vi "HXG2_SAVE Config File Values.vi"(8 "error in":errorcluster, 9 "BoolSelecOut":T1, 10 "AIR-GLY Cluster":T2 {"Liq Cluster"."Liq TEMP %" min=0.0 max=100.0 step=1.0 format="%#.1f"; "Liq Cluster"."Liq FLOW %" min=0.0 max=100.0 step=1.0 format="%#.1f"; "Liq Cluster"."TLiq °F" min=40.0 max=180.0 step=1.0 format="%#.1f"; "Liq Cluster"."Mdot lbm/hr" min=0.0 max=1000.0 step=1.0 format="%#.1f"; "Air Cluster"."Air TEMP %" min=0.0 max=100.0 step=1.0 format="%#.1f"; "Air Cluster"."Air FLOW %" min=0.0 max=100.0 step=1.0 format="%#.1f"; "Air Cluster"."Tair  °F" min=-5.0 max=100.0 step=1.0 format="%#.1f"; "Air Cluster"."CFMs" min=0.0 max=200.0 step=1.0 format="%#.1f"}) -> (0 "error out":errorcluster)   [LabVIEW 2012]
uses:
  Controls/HXG2_AirGly-Cluster.ctl
  Controls/UI/HXG2_UI_ControlSetAir.ctl
  Controls/UI/HXG2_UI_ControlSetGly.ctl
  Controls/HXG2_BooleanSelections.ctl
  <vilib>/Utility/file.llb/Write To Spreadsheet File (DBL).vi
panel:
  out "size(s)":i32
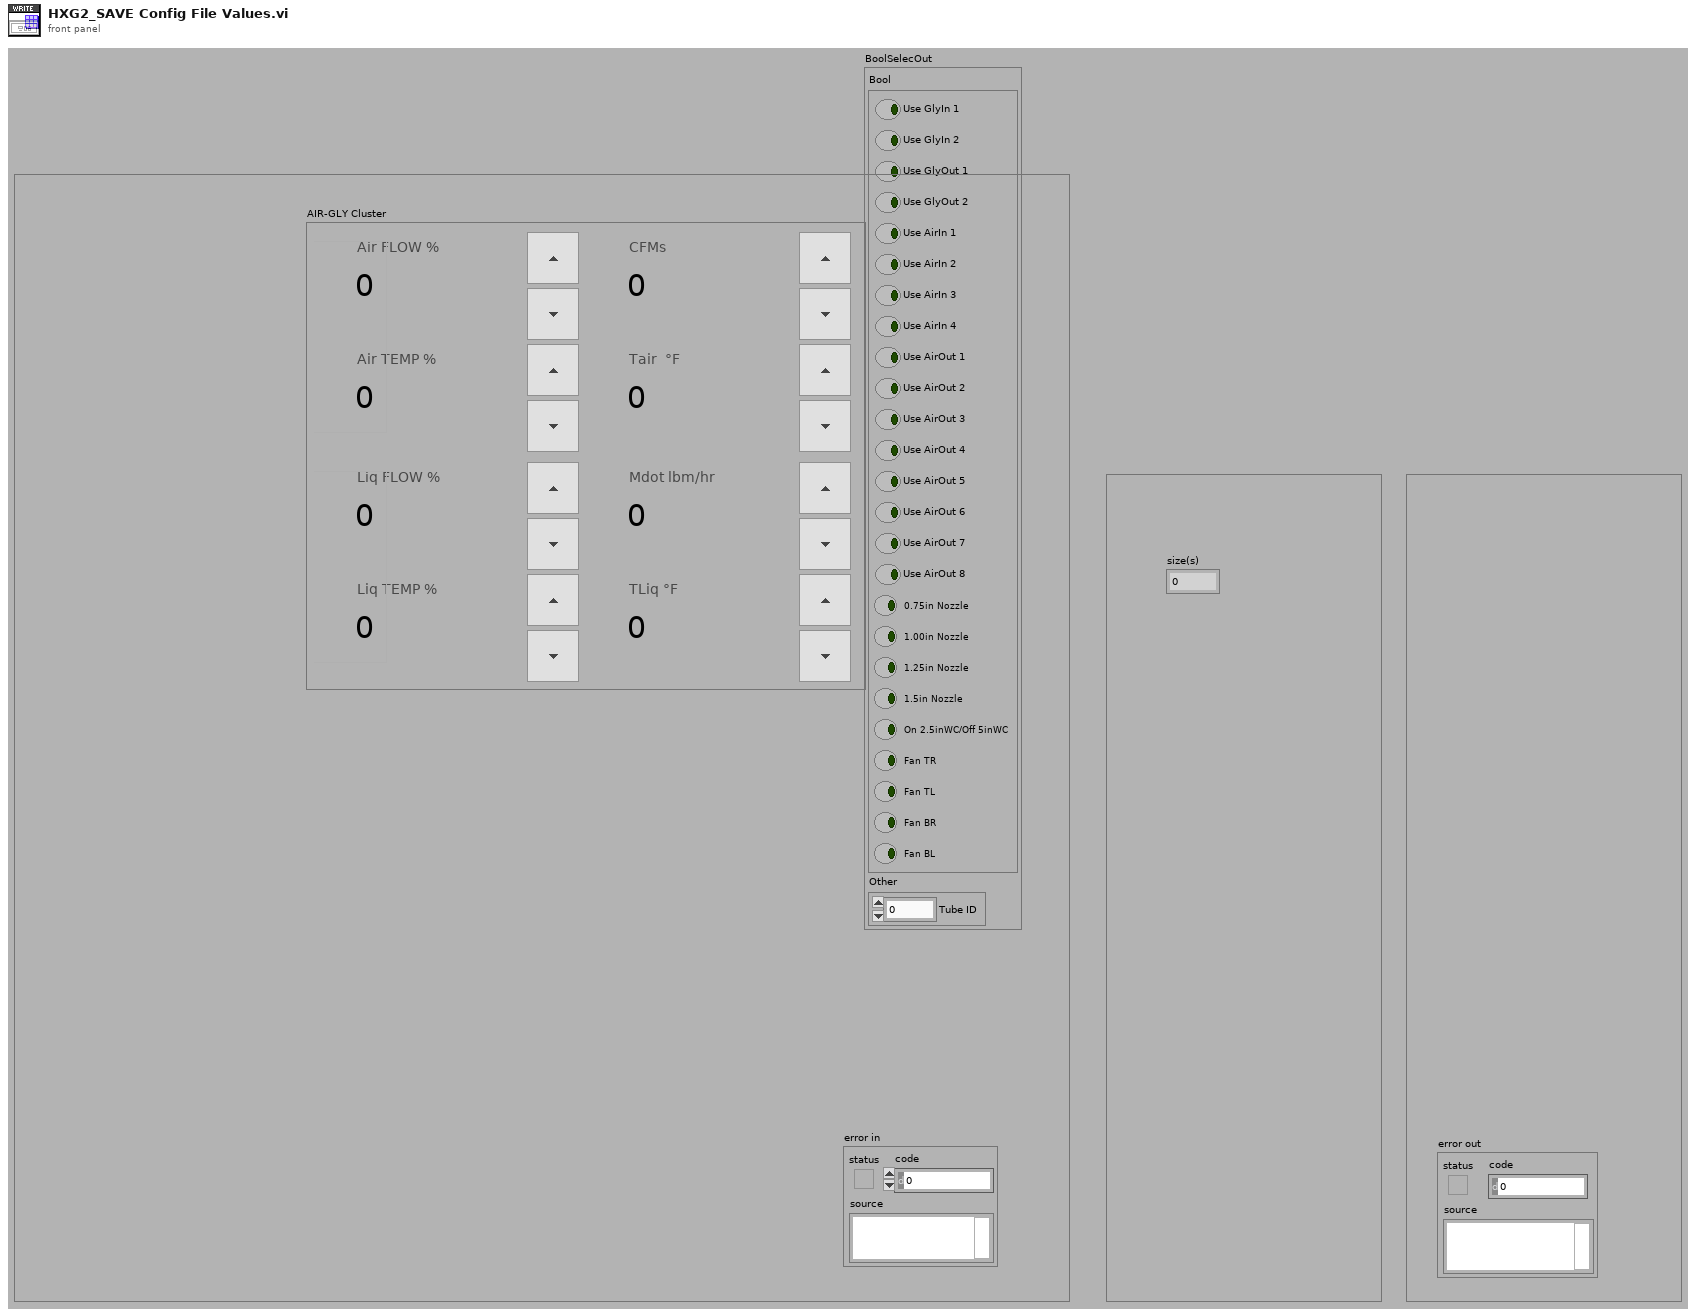
[diagram p1: front panel]
types:
  T1 = typedef "HXG2_BooleanSelections.ctl" = cluster{"Bool":cluster{"Use GlyIn 1":bool, "Use GlyIn 2":bool, "Use GlyOut 1":bool, "Use GlyOut 2":bool, "Use AirIn 1":bool, "Use AirIn 2":bool, "Use AirIn 3":bool, "Use AirIn 4":bool, "Use AirOut 1":bool, "Use AirOut 2":bool, "Use AirOut 3":bool, "Use AirOut 4":bool, "Use AirOut 5":bool, "Use AirOut 6":bool, "Use AirOut 7":bool, "Use AirOut 8":bool, "0.75in Nozzle":bool, "1.00in Nozzle":bool, "1.25in Nozzle":bool, "1.5in Nozzle":bool, "On 2.5inWC/Off 5inWC":bool, "Fan TR":bool, "Fan TL":bool, "Fan BR":bool, "Fan BL":bool}, "Other":cluster{"Tube ID":dbl}}
  T2 = typedef "HXG2_AirGly-Cluster.ctl" = cluster{"Air Cluster":T3, "Liq Cluster":T4}
  T3 = typedef "HXG2_UI_ControlSetAir.ctl" = cluster{"Air FLOW %":dbl, "Air TEMP % ":dbl, "CFMs":dbl, "Tair  °F":dbl}
  T4 = typedef "HXG2_UI_ControlSetGly.ctl" = cluster{"Liq FLOW %":dbl, "Liq TEMP % ":dbl, "Mdot lbm/hr":dbl, "TLiq °F":dbl}
  T5 = cluster{"Use GlyIn 1":bool, "Use GlyIn 2":bool, "Use GlyOut 1":bool, "Use GlyOut 2":bool, "Use AirIn 1":bool, "Use AirIn 2":bool, "Use AirIn 3":bool, "Use AirIn 4":bool, "Use AirOut 1":bool, "Use AirOut 2":bool, "Use AirOut 3":bool, "Use AirOut 4":bool, "Use AirOut 5":bool, "Use AirOut 6":bool, "Use AirOut 7":bool, "Use AirOut 8":bool, "0.75in Nozzle":bool, "1.00in Nozzle":bool, "1.25in Nozzle":bool, "1.5in Nozzle":bool, "On 2.5inWC/Off 5inWC":bool, "Fan TR":bool, "Fan TL":bool, "Fan BR":bool, "Fan BL":bool}
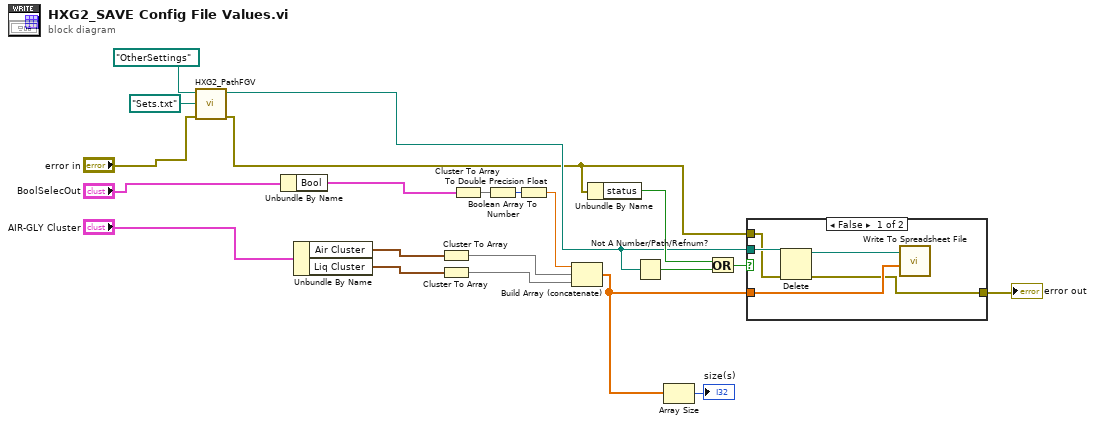
[diagram p0: block diagram]
diagram:
  n1 = call "HXG2_PathFGV.vi"("error in (no error)"="error in", "File Name"=path "Sets.txt", "Folder Name"=path "OtherSettings") -> ("error out"=w1:errorcluster, "File path"=w3:path)  [unwired: 5 in, 2 out]
  n2 = Unbundle By Name("BoolSelecOut") -> ("Bool"=w15:T5)
  n3 = Unbundle By Name("AIR-GLY Cluster") -> ("Air Cluster"=w13:T3, "Liq Cluster"=w12:T4)
  n4 = Cluster To Array(cluster=w13) -> (array=w10:dbl[])
  n5 = Cluster To Array(cluster=w12) -> (array=w11:dbl[])
  n6 = Cluster To Array(cluster=w15) -> (array=w19:bool[])
  n7 = Boolean Array To Number(Boolean array=w19) -> (number=w21:u32)
  n8 = To Double Precision Float(number=w21) -> (double precision float=w20:dbl)
  n9 = Build Array (concatenate)(w20, w10, w11) -> (w9:dbl[])
  n10 = Unbundle By Name(w1) -> ("status"=w6:bool)
  n11 = Not A Number/Path/Refnum?(number/path/refnum=w3) -> (NaN/Path/Refnum?=w7:bool)
  n12 = Array Size(array=w9) -> (size(s)=→"size(s)":i32)
  n13 = Or(x=w6, y=w7) -> (x .or. y?=w18:bool)
  n14 = case shown="False" w18 {
    tunnel: w9 -> [w26 _]
    tunnel: w3 -> [w25 _]
    tunnel: w1 -> [w23 w27]
    tunnel: [w22 w27] -> w14
    frame False {
      n15 = Delete(path (use dialog)=w25, error in=w23) -> (deleted path=w24:path, error out=w22:errorcluster)  [unwired: 4 out]
      n16 = call-poly <vilib>:"Write To Spreadsheet File.vi"("1D data"=w26, "file path (dialog if empty)"=w24) -> ()  [unwired: 4 in, 3 out]
    }
    frame True {
    }
  }
  "error out" <- w14
